vi "UserValidationCheck.vi"() -> ()   [LabVIEW 2024]
panel:
  out "FoundUserName":string
  out "Match FOund?":bool
  in  "Password":string
  in  "UserName":string
  out "error out":errorcluster
  in  "error in":errorcluster
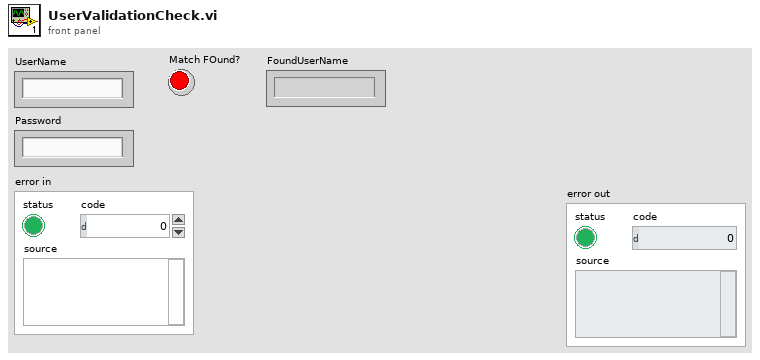
[diagram p1: front panel]
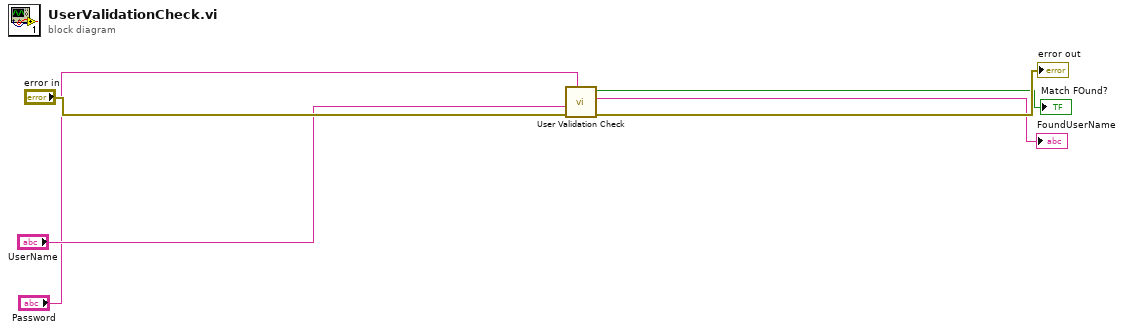
[diagram p0: block diagram]
diagram:
  n1 = call "User Validation Check.vi"("Password"="Password", "error in (no error)"="error in", "UserName"="UserName") -> ("error out"=→"error out":errorcluster, "String"=→"FoundUserName":string, "Boolean"=→"Match FOund?":bool)  [unwired: 6 in]
